vi "test-discretization-14.vi"(8 "error in (no error)":errorcluster) -> (0 "error out":errorcluster, 3 "All Tests Passed":bool)   [LabVIEW 2019]
uses:
  <vilib>/Analysis/Matrix/Datatypes/RealMatrix.ctl
  <vilib>/Analysis/baseanly.llb/Real A x B.vi
  <vilib>/Rock Robotics/WPI/ThirdParty/JAS_Junk/TrajLib/MatBuilder_Create.vi
  <vilib>/Rock Robotics/WPI/ThirdParty/JAS_Junk/TrajLib/MatrixHelper_CoerceSize.vi
  <vilib>/Rock Robotics/WPI/ThirdParty/JAS_Junk/TrajLib/Matrix_Exp.vi
  <vilib>/Rock Robotics/WPI/ThirdParty/JAS_Junk/TrajLib/Matrix_AssignBlock.vi
  <vilib>/Rock Robotics/WPI/ThirdParty/JAS_Junk/TrajLib/Matrix_ExtractFrom.vi
  <vilib>/Analysis/7linalg.llb/Transpose Matrix.vi
  <vilib>/Analysis/7linalg.llb/Real Transpose Matrix.vi
  <vilib>/Rock Robotics/WPI/ThirdParty/JAS_Junk/TrajLib/Matrix_Ident.vi
  <vilib>/Analysis/7linalg.llb/Matrix Exp.vi
  <vilib>/Analysis/7linalg.llb/Real Matrix Exp.vi
  <vilib>/Analysis/Matrix/Numeric/Multiply/Multiply.vi
  <vilib>/Analysis/Matrix/Numeric/Multiply/Multiply - RM,R.vi
  <vilib>/Analysis/7linalg.llb/Create Special Matrix.vi
  <vilib>/Analysis/7linalg.llb/Create Special Real Matrix.vi
  <vilib>/Analysis/Matrix/Numeric/Add/Add - RM,RM.vi
  <vilib>/Analysis/Matrix/Comparison/Equal/Equal - RM,RM.vi
  <vilib>/Rock Robotics/WPI/ThirdParty/JAS_Junk/TrajLib/Trajectory_Library.lvlib
  <vilib>/Analysis/NI_AALBase.lvlib
  <vilib>/Analysis/Matrix/NI_Matrix.lvlib
panel:
  out "X1Discrete 11":T1
  out "DiscB  11":T1
  out "Passed 11":bool
  out "DiscA  11":T1
  out "Passed 10":bool
  out "DiscA  10":T1
  out "Passed 16":bool
  out "DiscR  16":T1
  out "A+B Should be":T1
  out "A + B":T1
  out "Test x passed":bool
  out "Test 3 passed":bool
  out "Test Passed 2":bool
  out "Test Passed 1":bool
  out "Test Passed 0":bool
  out "AQ Passed":bool
  out "AQ - DiscQ":T1
  out "AQ - DiscA":T1
  out "AB-Taylor-Passed":bool
  out "ABTaylor-DiscB":T1
  out "ABTaylor - DiscA":T1
  out "AB-passed":bool
  out "AB-DiscB":T1
  out "AB - DiscA":T1
  out "x1-Disc":T1
  out "DiscA Error":bool
  out "DiscA":T1
  out "Cost Mat":T1
  out "CoVar Mat":T1
  # "1.0,   0.0,    0.0\n\n0.0,     4.0,   0.0, ;\n\n0.0,     0.0,  9.0;"
  # "1.0,      0.0,      0.0, \n\n0.0,   1.0 / 4.0,   0.0, \n\n0.0,       0.0,      1.0 / 9.0,"
  # "VecBuilder.fill(\n          x0.get(0, 0) + 1.0 * x0.get(1, 0), \n          x0.get(1, 0));"
  # "2,\n1"
  # "x0.get(0, 0) + x0.get(1, 0) + 0.5 * u.get(0, 0), \n\nx0.get(0, 0) + u.get(0, 0))"
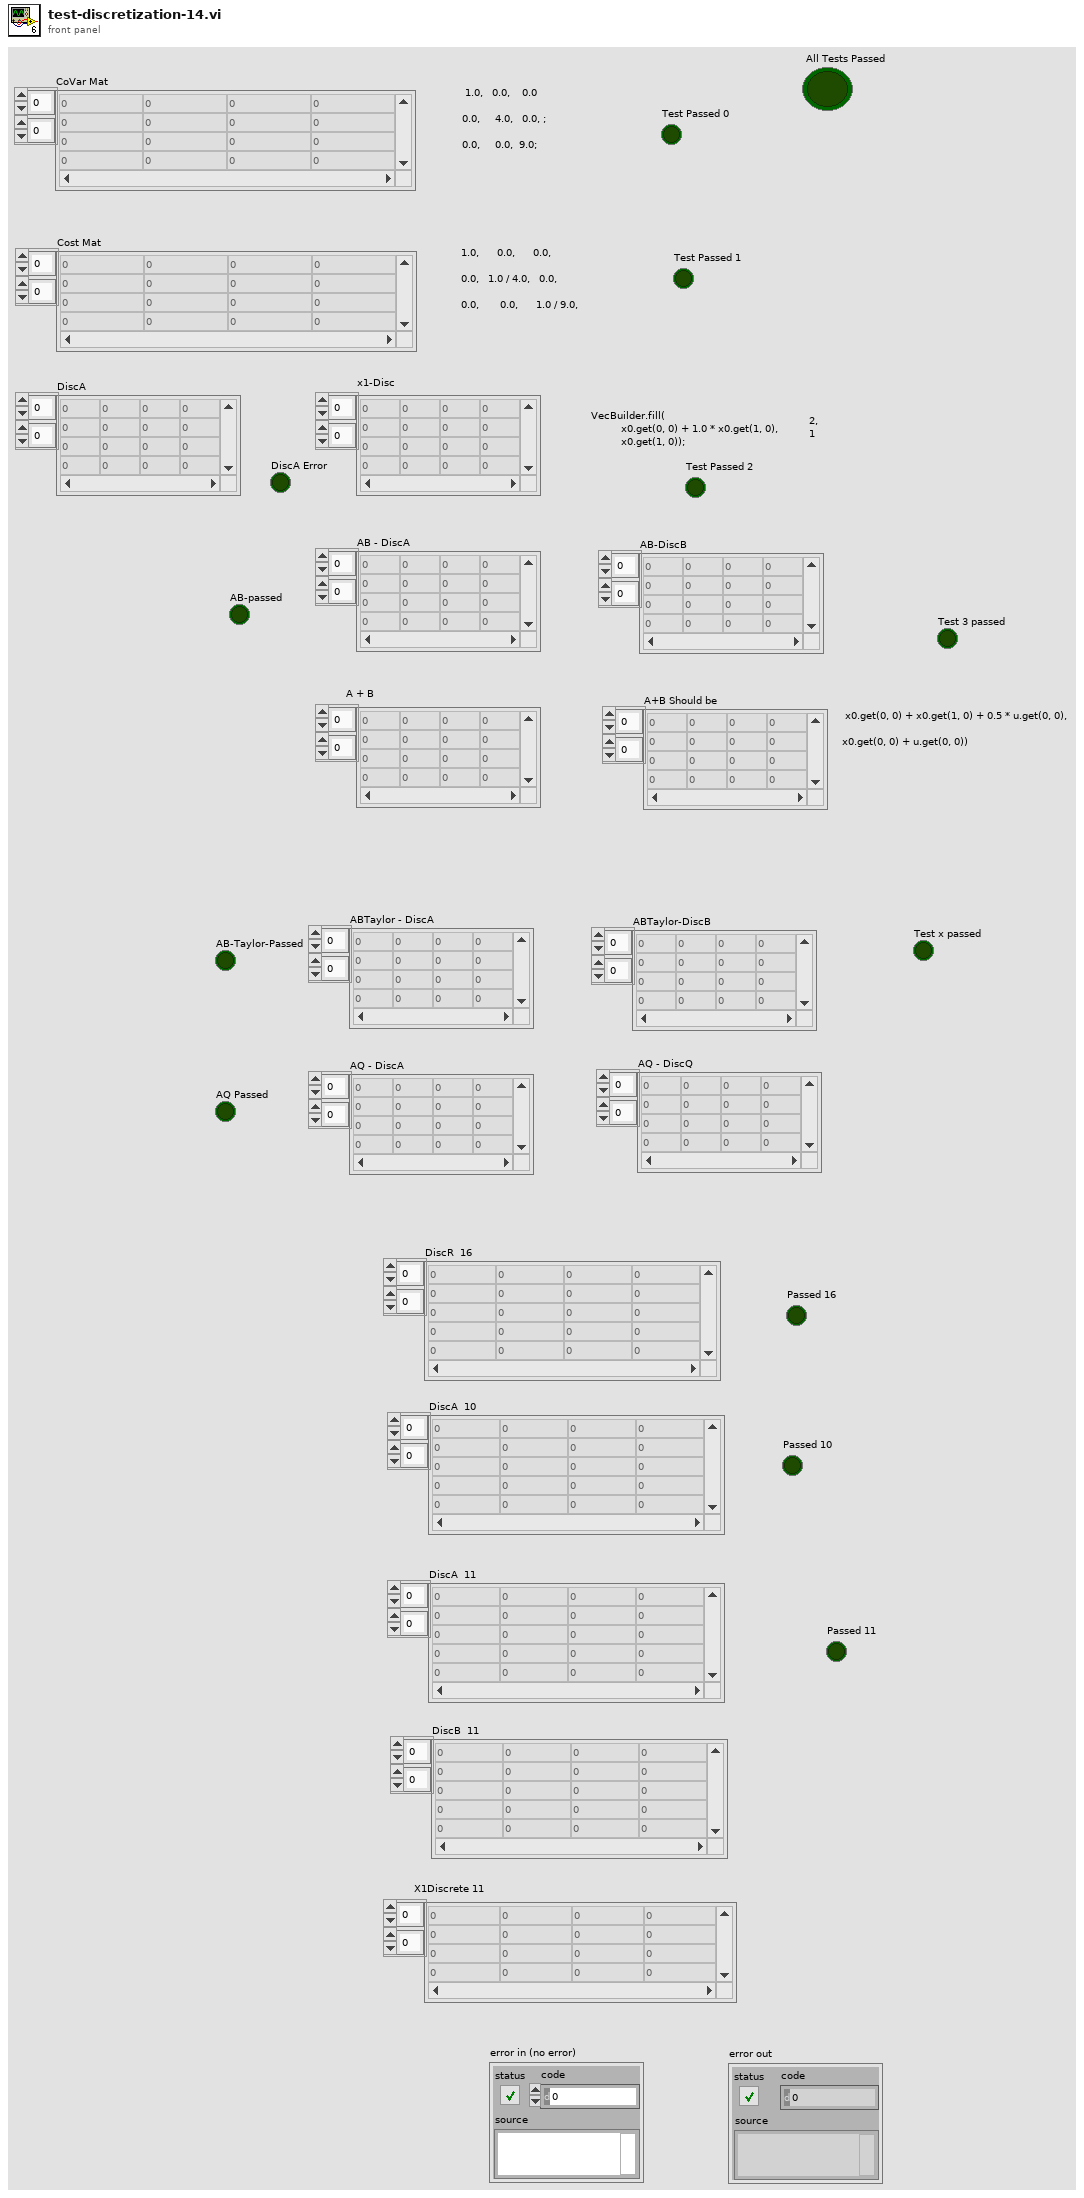
[diagram p1: front panel]
types:
  T1 = typedef "NI_Matrix.lvlib/RealMatrix.ctl" = dbl[][]
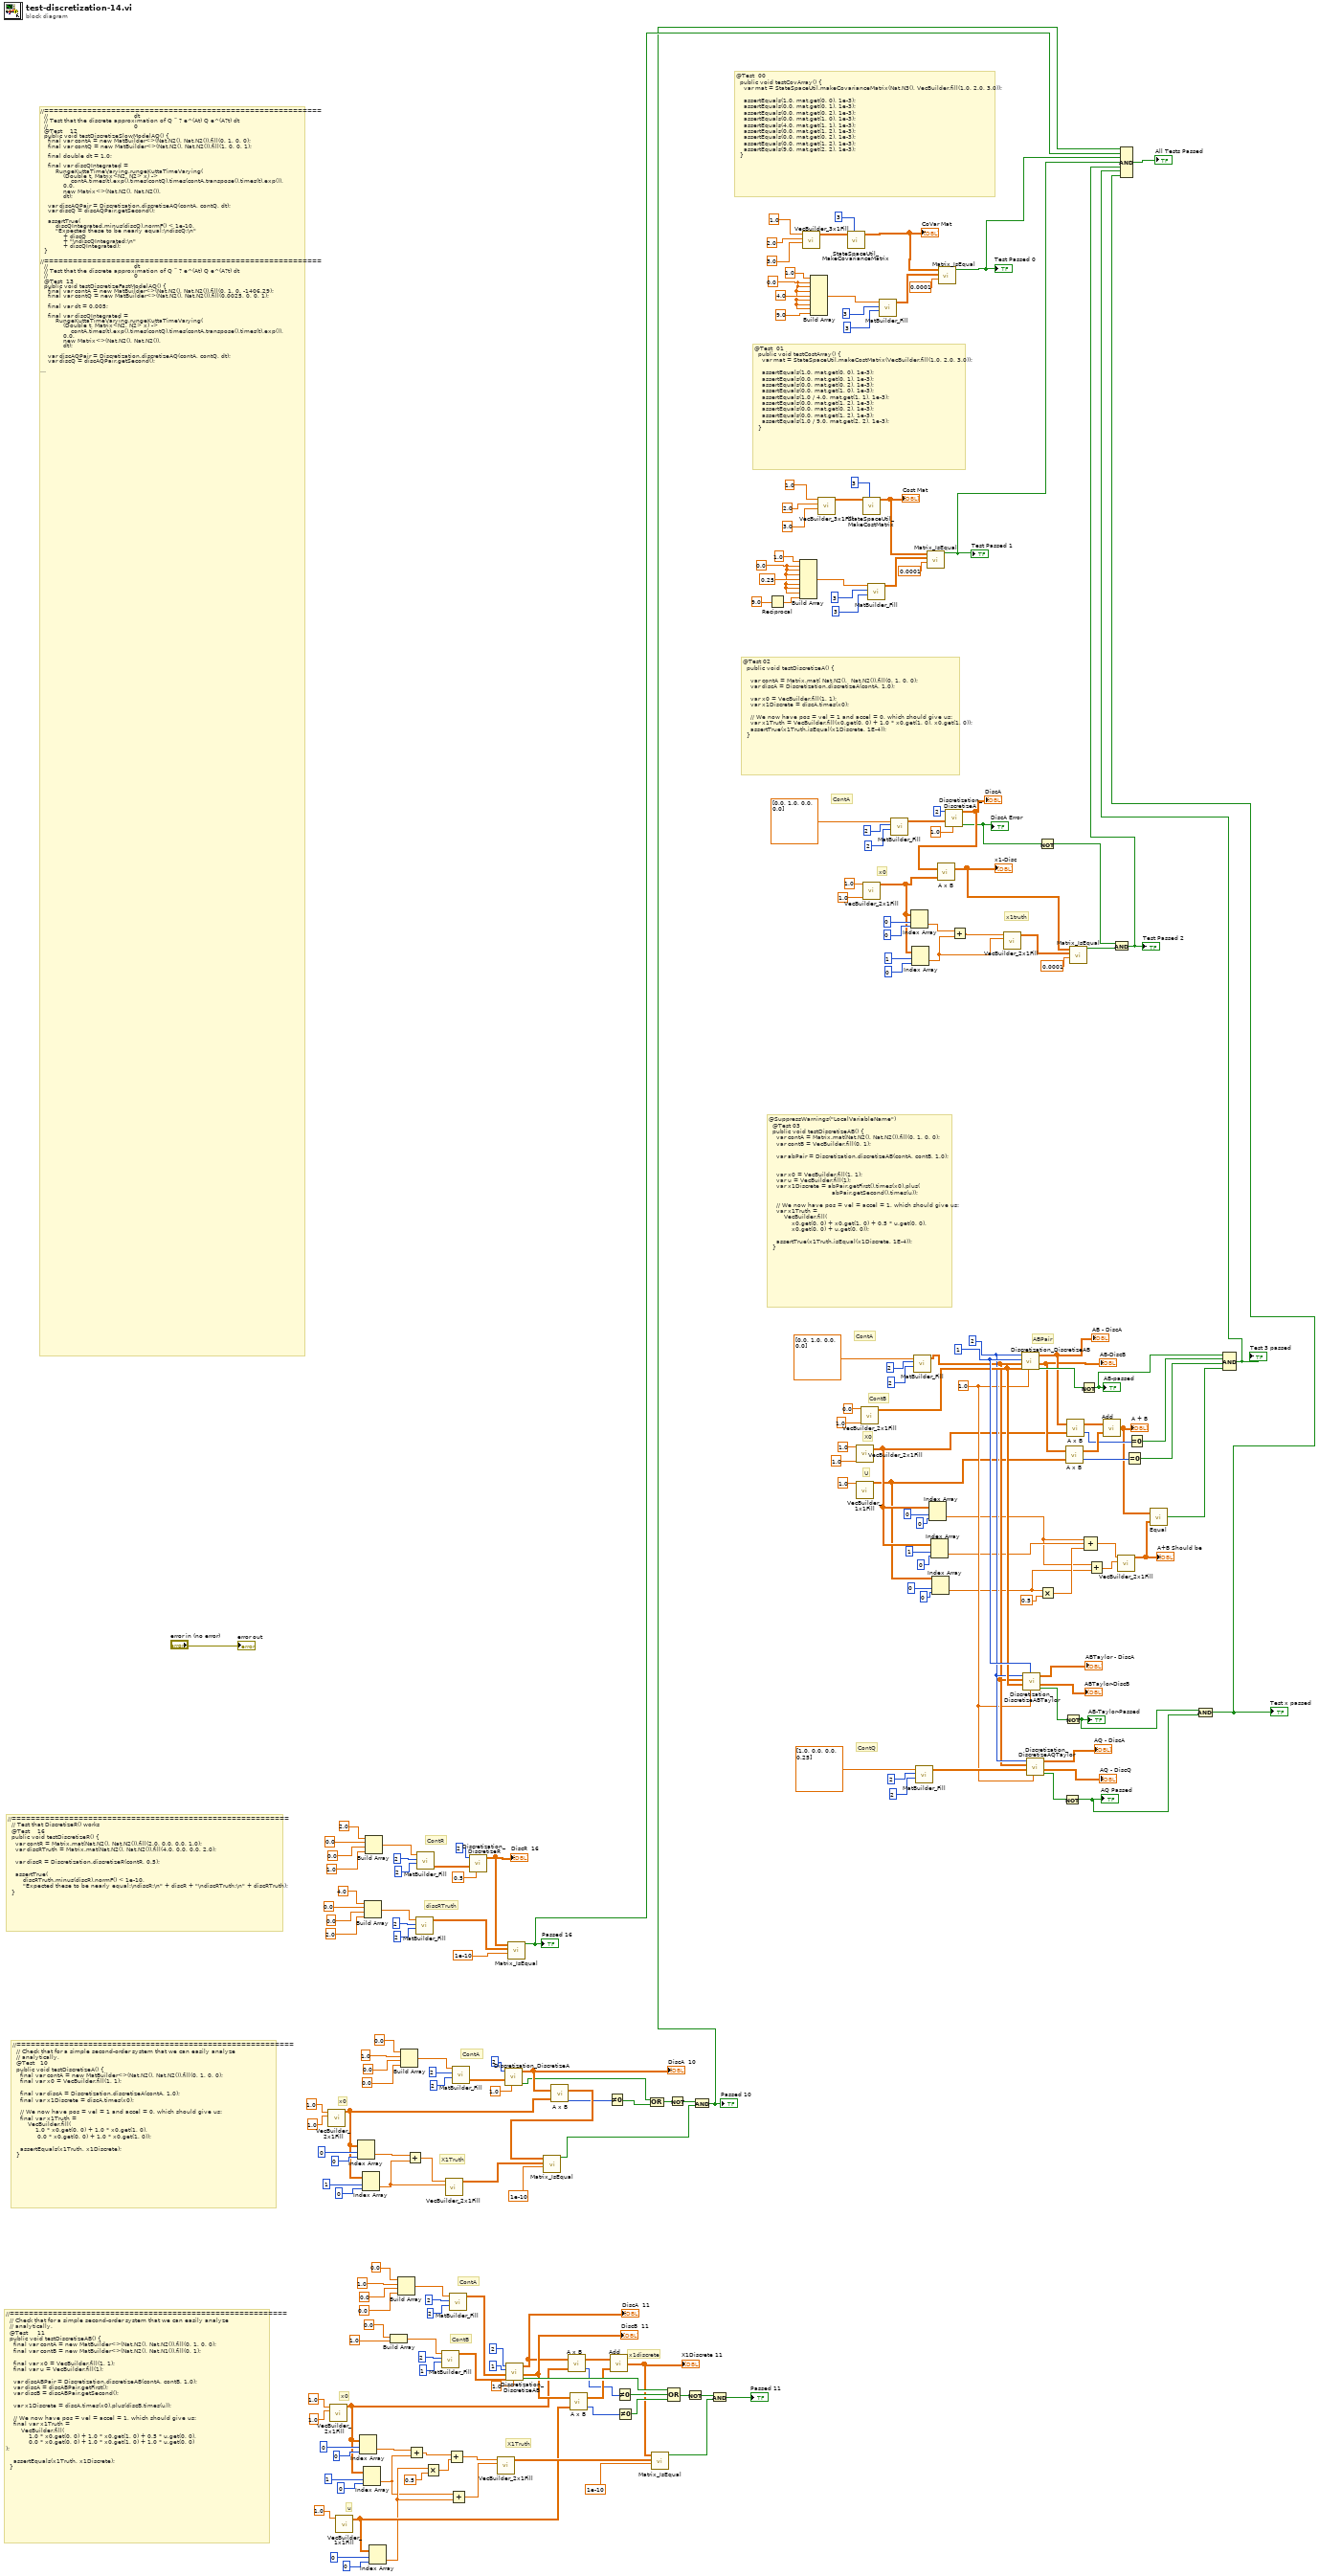
[diagram p0: block diagram]
diagram:
  w166 = 0.0 ("element")
  w176 = 0.0 ("element")
  w184 = 1.0 ("dT_Seconds")
  w194 = 1 ("Inputs")
  w187 = 2 ("States")
  # "x1discrete"
  # "u"
  # "ContB"
  # "X1Truth"
  # "x0"
  # "ContA"
  # "//==========================================================\n  // Check that for a simple second-order system that we can easily analyze\n  // analytically,\n  @Test     11\n  public void testDiscretizeAB() {\n    final var contA = new MatBuilder<>(Nat.N2(), Nat.N2()).fill(0, 1, 0, 0);\n    final var contB = new MatBuilder<>(Nat.N2(), Nat.N1()).fill(0, 1);\n\n    final var x0 = VecBuilder.fill(1, 1);\n    final var u = VecBuilder.fill(1);\n\n    var discABPair = Discretization.discretizeAB(contA, contB, 1.0);\n    var discA = discABPair.getFirst();\n    var discB = discABPair.getSecond();\n\n    var x1Discrete = discA.times(x0).plus(discB.times(u));\n\n    // We now have pos = vel = accel = 1, which should give us:\n    final var x1Truth =\n        VecBuilder.fill(\n            1.0 * x0.get(0, 0) + 1.0 * x0.get(1, 0) + 0.5 * u.get(0, 0),\n            0.0 * x0.get(0, 0) + 1.0 * x0.get(1, 0) + 1.0 * u.get(0, 0)\n);\n\n    assertEquals(x1Truth, x1Discrete);\n  }"
  # "X1Truth"
  # "x0"
  # "ContA"
  # "//==========================================================\n  // Check that for a simple second-order system that we can easily analyze\n  // analytically,\n  @Test   10\n  public void testDiscretizeA() {\n    final var contA = new MatBuilder<>(Nat.N2(), Nat.N2()).fill(0, 1, 0, 0);\n    final var x0 = VecBuilder.fill(1, 1);\n\n    final var discA = Discretization.discretizeA(contA, 1.0);\n    final var x1Discrete = discA.times(x0);\n\n    // We now have pos = vel = 1 and accel = 0, which should give us:\n    final var x1Truth =\n        VecBuilder.fill(\n            1.0 * x0.get(0, 0) + 1.0 * x0.get(1, 0), \n             0.0 * x0.get(0, 0) + 1.0 * x0.get(1, 0));\n\n    assertEquals(x1Truth, x1Discrete);\n  }"
  # "discRTruth"
  # "ContR"
  # "//==========================================================\n  // Test that DiscretizeR() works\n  @Test    16\n  public void testDiscretizeR() {\n    var contR = Matrix.mat(Nat.N2(), Nat.N2()).fill(2.0, 0.0, 0.0, 1.0);\n    var discRTruth = Matrix.mat(Nat.N2(), Nat.N2()).fill(4.0, 0.0, 0.0, 2.0);\n\n    var discR = Discretization.discretizeR(contR, 0.5);\n\n    assertTrue(\n        discRTruth.minus(discR).normF() < 1e-10,\n        \"Expected these to be nearly equal:\\ndiscR:\\n\" + discR + \"\\ndiscRTruth:\\n\" + discRTruth);\n  }"
  # "//==========================================================\n  //                                             dt\n  // Test that the discrete approximation of Q ˜ ? e^(At) Q e^(A?t) dt\n  //                                             0\n  @Test    12\n  public void testDiscretizeSlowModelAQ() {\n    final var contA = new MatBuilder<>(Nat.N2(), Nat.N2()).fill(0, 1, 0, 0);\n    final var contQ = new MatBuilder<>(Nat.N2(), Nat.N2()).fill(1, 0, 0, 1);\n\n    final double dt = 1.0;\n\n    final var discQIntegrated =\n        RungeKuttaTimeVarying.rungeKuttaTimeVarying(\n            (Double t, Matrix<N2, N2> x) ->\n                contA.times(t).exp().times(contQ).times(contA.transpose().times(t).exp()),\n            0.0,\n            new Matrix<>(Nat.N2(), Nat.N2()),\n            dt);\n\n    var discAQPair = Discretization.discretizeAQ(contA, contQ, dt);\n    var discQ = discAQPair.getSecond();\n\n    assertTrue(\n        discQIntegrated.minus(discQ).normF() < 1e-10,\n        \"Expected these to be nearly equal:\\ndiscQ:\\n\"\n            + discQ\n            + \"\\ndiscQIntegrated:\\n\"\n            + discQIntegrated);\n  }\n\n//==========================================================\n  //                                             dt\n  // Test that the discrete approximation of Q ˜ ? e^(At) Q e^(A?t) dt\n  //                                             0\n  @Test  13\n  public void testDiscretizeFastModelAQ() {\n    final var contA = new MatBuilder<>(Nat.N2(), Nat.N2()).fill(0, 1, 0, -1406.29);\n    final var contQ = new MatBuilder<>(Nat.N2(), Nat.N2()).fill(0.0025, 0, 0, 1);\n\n    final var dt = 0.005;\n\n    final var discQIntegrated =\n        RungeKuttaTimeVarying.rungeKuttaTimeVarying(\n            (Double t, Matrix<N2, N2> x) ->\n                contA.times(t).exp().times(contQ).times(contA.transpose().times(t).exp()),\n            0.0,\n            new Matrix<>(Nat.N2(), Nat.N2()),\n            dt);\n\n    var discAQPair = Discretization.discretizeAQ(contA, contQ, dt);\n    var discQ = discAQPair.getSecond();\n\n    assertTrue(\n        discQIntegrated.minus(discQ).normF() < 1e-3,\n        \"Expected these to be nearly equal:\\ndiscQ:\\n\"\n            + discQ\n            + \"\\ndiscQIntegrated:\\n\"\n            + discQIntegrated);\n  }\n\n//==========================================================\n  // Test that the Taylor series discretization produces nearly identical results.\n  @Test  14\n  public void testDiscretizeSlowModelAQTaylor() {\n    final var contA = new MatBuilder<>(Nat.N2(), Nat.N2()).fill(0, 1, 0, 0);\n    final var contQ = new MatBuilder<>(Nat.N2(), Nat.N2()).fill(1, 0, 0, 1);\n\n    final var dt = 1.0;\n\n    // Continuous Q should be positive semidefinite\n    final var esCont = contQ.getStorage().eig();\n    for (int i = 0; i < contQ.getNumRows(); ++i) {\n      assertTrue(esCont.getEigenvalue(i).real >= 0);\n    }\n\n    final var discQIntegrated =\n        RungeKuttaTimeVarying.rungeKuttaTimeVarying(\n            (Double t, Matrix<N2, N2> x) ->\n                contA.times(t).exp().times(contQ).times(contA.transpose().times(t).exp()),\n            0.0,\n            new Matrix<>(Nat.N2(), Nat.N2()),\n            dt);\n\n    var discA = Discretization.discretizeA(contA, dt);\n\n    var discAQPair = Discretization.discretizeAQ(contA, contQ, dt);\n    var discATaylor = discAQPair.getFirst();\n    var discQTaylor = discAQPair.getSecond();\n\n    assertTrue(\n        discQIntegrated.minus(discQTaylor).normF() < 1e-10,\n        \"Expected these to be nearly equal:\\ndiscQTaylor:\\n\"\n            + discQTaylor\n            + \"\\ndiscQIntegrated:\\n\"\n            + discQIntegrated);\n    assertTrue(discA.minus(discATaylor).normF() < 1e-10);\n\n    // Discrete Q should be positive semidefinite\n    final var esDisc = discQTaylor.getStorage().eig();\n    for (int i = 0; i < discQTaylor.getNumRows(); ++i) {\n      assertTrue(esDisc.getEigenvalue(i).real >= 0);\n    }\n  }\n\n//==========================================================\n  // Test that the Taylor series discretization produces nearly identical results.\n  @Test  15\n  public void testDiscretizeFastModelAQTaylor() {\n    final var contA = new MatBuilder<>(Nat.N2(), Nat.N2()).fill(0, 1, 0, -1500);\n    final var contQ = new MatBuilder<>(Nat.N2(), Nat.N2()).fill(0.0025, 0, 0, 1);\n\n    final var dt = 0.005;\n\n    // Continuous Q should be positive semidefinite\n    final var esCont = contQ.getStorage().eig();\n    for (int i = 0; i < contQ.getNumRows(); ++i) {\n      assertTrue(esCont.getEigenvalue(i).real >= 0);\n    }\n\n    final var discQIntegrated =\n        RungeKuttaTimeVarying.rungeKuttaTimeVarying(\n            (Double t, Matrix<N2, N2> x) ->\n                contA.times(t).exp().times(contQ).times(contA.transpose().times(t).exp()),\n            0.0,\n            new Matrix<>(Nat.N2(), Nat.N2()),\n            dt);\n\n    var discA = Discretization.discretizeA(contA, dt);\n\n    var discAQPair = Discretization.discretizeAQ(contA, contQ, dt);\n    var discATaylor = discAQPair.getFirst();\n    var discQTaylor = discAQPair.getSecond();\n\n    assertTrue(\n        discQIntegrated.minus(discQTaylor).normF() < 1e-3,\n        \"Expected these to be nearly equal:\\ndiscQTaylor:\\n\"\n            + discQTaylor\n            + \"\\ndiscQIntegrated:\\n\"\n            + discQIntegrated);\n    assertTrue(discA.minus(discATaylor).normF() < 1e-10);\n\n    // Discrete Q should be positive semidefinite\n    final var esDisc = discQTaylor.getStorage().eig();\n    for (int i = 0; i < discQTaylor.getNumRows(); ++i) {\n      assertTrue(esDisc.getEigenvalue(i).real >= 0);\n    }\n  }\n\n}"
  # "U"
  # "X0"
  # "ContB"
  # "ABPair"
  # "x1truth"
  # "x0"
  # "ContQ"
  # "ContA"
  # "@SuppressWarnings(\"LocalVariableName\")\n  @Test 03\n  public void testDiscretizeAB() {\n    var contA = Matrix.mat(Nat.N2(), Nat.N2()).fill(0, 1, 0, 0);\n    var contB = VecBuilder.fill(0, 1);\n\n    var abPair = Discretization.discretizeAB(contA, contB, 1.0);\n\n\n    var x0 = VecBuilder.fill(1, 1);\n    var u = VecBuilder.fill(1);\n    var x1Discrete = abPair.getFirst().times(x0).plus(\n                                 abPair.getSecond().times(u));\n\n    // We now have pos = vel = accel = 1, which should give us:\n    var x1Truth =\n        VecBuilder.fill(\n            x0.get(0, 0) + x0.get(1, 0) + 0.5 * u.get(0, 0), \n            x0.get(0, 0) + u.get(0, 0));\n\n    assertTrue(x1Truth.isEqual(x1Discrete, 1E-4));\n  }"
  # "ContA"
  # "@Test 02\n  public void testDiscretizeA() {\n\n    var contA = Matrix.mat( Nat.N2(),  Nat.N2()).fill(0, 1, 0, 0);\n    var discA = Discretization.discretizeA(contA, 1.0);\n\n    var x0 = VecBuilder.fill(1, 1);\n    var x1Discrete = discA.times(x0);\n\n    // We now have pos = vel = 1 and accel = 0, which should give us:\n    var x1Truth = VecBuilder.fill(x0.get(0, 0) + 1.0 * x0.get(1, 0), x0.get(1, 0));\n    assertTrue(x1Truth.isEqual(x1Discrete, 1E-4));\n  }"
  # "@Test  01\n  public void testCostArray() {\n    var mat = StateSpaceUtil.makeCostMatrix(VecBuilder.fill(1.0, 2.0, 3.0));\n\n    assertEquals(1.0, mat.get(0, 0), 1e-3);\n    assertEquals(0.0, mat.get(0, 1), 1e-3);\n    assertEquals(0.0, mat.get(0, 2), 1e-3);\n    assertEquals(0.0, mat.get(1, 0), 1e-3);\n    assertEquals(1.0 / 4.0, mat.get(1, 1), 1e-3);\n    assertEquals(0.0, mat.get(1, 2), 1e-3);\n    assertEquals(0.0, mat.get(0, 2), 1e-3);\n    assertEquals(0.0, mat.get(1, 2), 1e-3);\n    assertEquals(1.0 / 9.0, mat.get(2, 2), 1e-3);\n  }"
  # "@Test  00\n  public void testCovArray() {\n    var mat = StateSpaceUtil.makeCovarianceMatrix(Nat.N3(), VecBuilder.fill(1.0, 2.0, 3.0));\n\n    assertEquals(1.0, mat.get(0, 0), 1e-3);\n    assertEquals(0.0, mat.get(0, 1), 1e-3);\n    assertEquals(0.0, mat.get(0, 2), 1e-3);\n    assertEquals(0.0, mat.get(1, 0), 1e-3);\n    assertEquals(4.0, mat.get(1, 1), 1e-3);\n    assertEquals(0.0, mat.get(1, 2), 1e-3);\n    assertEquals(0.0, mat.get(0, 2), 1e-3);\n    assertEquals(0.0, mat.get(1, 2), 1e-3);\n    assertEquals(9.0, mat.get(2, 2), 1e-3);\n  }"
  n1 = call <vilib>:"VecBuilder_2x1Fill.vi"("R1"=1.0, "R0"=1.0) -> ("output matrix"=w66:T1)  [unwired: 9 in]
  n2 = call <vilib>:"VecBuilder_2x1Fill.vi"("R1"=1.0, "R0"=1.0) -> ("output matrix"=w19:T1)  [unwired: 9 in]
  n3 = call <vilib>:"VecBuilder_1x1Fill.vi"("R0_C0"=1.0 ("R0")) -> ("output matrix"=w10:T1)  [unwired: 10 in]
  n4 = Index Array(array=w66, index (row)=0, index (col)=0) -> (element=w63:dbl)
  n5 = Index Array(array=w19, index (row)=0, index (col)=0) -> (element=w37:dbl)
  n6 = Index Array(array=w66, index (row)=1, index (col)=0) -> (element=w62:dbl)
  n7 = Index Array(array=w19, index (row)=1, index (col)=0) -> (element=w4:dbl)
  n8 = Build Array(4.0 ("element"), 0.0 ("element"), 0.0 ("element"), 2.0 ("element")) -> (w98:dbl[])
  n9 = Build Array(2.0 ("element"), 0.0 ("element"), 0.0 ("element"), 1.0 ("element")) -> (w105:dbl[])
  n10 = Index Array(array=w10, index (row)=0, index (col)=0) -> (element=w5:dbl)
  n11 = Build Array(0.0 ("element"), 1.0 ("element")) -> (w30:dbl[])
  n12 = Build Array(0.0 ("element"), 1.0 ("element"), 0.0 ("element"), 0.0 ("element")) -> (w54:dbl[])
  n13 = Build Array(0.0 ("element"), 1.0 ("element"), 0.0 ("element"), 0.0 ("element")) -> (w84:dbl[])
  n14 = Add(x=w63, y=w62) -> (x+y=w64:dbl)
  n15 = Add(x=w37, y=w4) -> (x+y=w7:dbl)
  n16 = call <vilib>:"MatBuilder_Fill.vi"("Columns"=2, "Rows"=2, "Value List"=w98) -> ("output matrix"=w87:T1)  [unwired: 8 in]
  n17 = call <vilib>:"MatBuilder_Fill.vi"("Columns"=2, "Rows"=2, "Value List"=w105) -> ("output matrix"=w90:T1)  [unwired: 8 in]
  n18 = Multiply(x=w5, y=0.5) -> (x*y=w8:dbl)
  n19 = call <vilib>:"MatBuilder_Fill.vi"("Columns"=1, "Rows"=2, "Value List"=w30) -> ("output matrix"=w24:T1)  [unwired: 8 in]
  n20 = call <vilib>:"VecBuilder_2x1Fill.vi"("R1"=w62, "R0"=w64) -> ("output matrix"=w65:T1)  [unwired: 9 in]
  n21 = Add(x=w7, y=w8) -> (x+y=w6:dbl)
  n22 = call <vilib>:"MatBuilder_Fill.vi"("Columns"=2, "Rows"=2, "Value List"=w54) -> ("output matrix"=w25:T1)  [unwired: 8 in]
  n23 = Add(x=w4, y=w5) -> (x+y=w3:dbl)
  n24 = call <vilib>:"MatBuilder_Fill.vi"("Columns"=2, "Rows"=2, "Value List"=w84) -> ("output matrix"=w76:T1)  [unwired: 8 in]
  n25 = call <vilib>:"Discretization_DiscretizeR.vi"("dT_Seconds"=0.5, "ContR"=w90, "Outputs"=2) -> ("DiscR"=w89:T1)  [unwired: 7 in, 1 out]
  "DiscR  16" <- w89
  n26 = call <vilib>:"VecBuilder_2x1Fill.vi"("R1"=w3, "R0"=w6) -> ("output matrix"=w38:T1)  [unwired: 9 in]
  n27 = call <vilib>:"Discretization_DiscretizeA.vi"("dT_Seconds"=1.0, "ContA"=w76, "States"=2 ("Outputs")) -> ("Error"=w59:bool, "DiscA"=w71:T1)  [unwired: 7 in]
  "DiscA  10" <- w71
  n28 = call <vilib>:"Discretization_DiscretizeAB.vi"("dT_Seconds"=1.0, "ContB"=w24, "ContA"=w25, "Inputs"=1, "States"=2 ("Outputs")) -> ("Error"=w36:bool, "DiscB"=w21:T1, "DiscA"=w20:T1)  [unwired: 4 in]
  "DiscA  11" <- w20
  "DiscB  11" <- w21
  n29 = call <vilib>:"Matrix_IsEqual.vi"("Tolerance"=1e-10, "other"=w87, "input matrix"=w89) -> ("Equal"=w85:bool)  [unwired: 8 in]
  "Passed 16" <- w85
  n30 = call-poly <vilib>:"A x B.vi"("B"=w66, "A"=w71) -> ("error"=w60:i32, "A x B"=w61:T1)
  n31 = call <vilib>:"Matrix_IsEqual.vi"("Tolerance"=1e-10, "other"=w65, "input matrix"=w61) -> ("Equal"=w55:bool)  [unwired: 8 in]
  n32 = call-poly <vilib>:"A x B.vi"("B"=w19, "A"=w20) -> ("error"=w15:i32, "A x B"=w18:T1)
  n33 = call-poly <vilib>:"A x B.vi"("B"=w10, "A"=w21) -> ("error"=w14:i32, "A x B"=w17:T1)
  n34 = Not Equal To 0?(x=w60) -> (x != 0?=w58:bool)
  n35 = call-poly <vilib>:"Add.vi"("Real Matrix B"=w17, "Real Matrix A"=w18) -> ("A + B"=w13:T1)
  "X1Discrete 11" <- w13
  n36 = Not Equal To 0?(x=w15) -> (x != 0?=w35:bool)
  n37 = Not Equal To 0?(x=w14) -> (x != 0?=w16:bool)
  n38 = Compound Arithmetic op=OR(w59, w58) -> (w57:bool)
  n39 = call <vilib>:"Matrix_IsEqual.vi"("Tolerance"=1e-10, "other"=w38, "input matrix"=w13) -> ("Equal"=w32:bool)  [unwired: 8 in]
  n40 = Compound Arithmetic op=OR(w36, w35, w16) -> (w34:bool)
  n41 = Not(x=w57) -> (.not. x?=w56:bool)
  n42 = Not(x=w34) -> (.not. x?=w33:bool)
  n43 = And(x=w56, y=w55) -> (x .and. y?=w2:bool)
  "Passed 10" <- w2
  n44 = And(x=w33, y=w32) -> (x .and. y?=→"Passed 11":bool)
  n45 = Reciprocal(x=9.0 ("element")) -> (1/x=w162:dbl)
  n46 = Build Array(1.0 ("element"), w166, w166, w166, 0.25 ("element"), w166, w166, w166, w162) -> (w169:dbl[])
  n47 = call <vilib>:"VecBuilder_3x1Fill.vi"("R2"=3.0, "R1"=2.0, "R0"=1.0) -> ("output matrix"=w215:T1)  [unwired: 8 in]
  n48 = Build Array(1.0 ("element"), w176, w176, w176, 4.0 ("element"), w176, w176, w176, 9.0 ("element")) -> (w179:dbl[])
  n49 = call <vilib>:"VecBuilder_3x1Fill.vi"("R2"=3.0, "R1"=2.0, "R0"=1.0) -> ("output matrix"=w210:T1)  [unwired: 8 in]
  n50 = call <vilib>:"StateSpaceUtil_MakeCovarianceMatrix.vi"("States"=3, "StdDevs"=w215) -> ("Covariance Matrix"=w174:T1)  [unwired: 8 in, 1 out]
  "CoVar Mat" <- w174
  n51 = call <vilib>:"VecBuilder_2x1Fill.vi"("R1"=1.0, "R0"=1.0 ("R0_C0")) -> ("output matrix"=w117:T1)  [unwired: 9 in]
  n52 = call <vilib>:"VecBuilder_1x1Fill.vi"("R0_C0"=1.0) -> ("output matrix"=w116:T1)  [unwired: 10 in]
  n53 = call <vilib>:"VecBuilder_2x1Fill.vi"("R1"=1.0, "R0"=0.0 ("R0_C0")) -> ("output matrix"=w193:T1)  [unwired: 9 in]
  n54 = call <vilib>:"StateSpaceUtil_MakeCostMatrix.vi"("States"=3, "Costs"=w210) -> ("Costs Matrix"=w161:T1)  [unwired: 8 in, 1 out]
  "Cost Mat" <- w161
  n55 = call <vilib>:"VecBuilder_2x1Fill.vi"("R1"=1.0, "R0"=1.0 ("R0_C0")) -> ("output matrix"=w155:T1)  [unwired: 9 in]
  n56 = call <vilib>:"MatBuilder_Fill.vi"("Columns"=3, "Rows"=3, "Value List"=w169) -> ("output matrix"=w165:T1)  [unwired: 8 in]
  n57 = call <vilib>:"MatBuilder_Fill.vi"("Columns"=3, "Rows"=3, "Value List"=w179) -> ("output matrix"=w173:T1)  [unwired: 8 in]
  n58 = call <vilib>:"MatBuilder_Fill.vi"("Columns"=2, "Rows"=2, "Value List"=dbl[] [0.0, 1.0, 0.0, 0.0]) -> ("output matrix"=w203:T1)  [unwired: 8 in]
  n59 = Index Array(array=w155, index (row)=0, index (col)=0) -> (element=w154:dbl)
  n60 = Index Array(array=w155, index (row)=1, index (col)=0) -> (element=w152:dbl)
  n61 = call <vilib>:"MatBuilder_Fill.vi"("Columns"=2, "Rows"=2, "Value List"=dbl[] [0.0, 1.0, 0.0, 0.0]) -> ("output matrix"=w186:T1)  [unwired: 8 in]
  n62 = call <vilib>:"MatBuilder_Fill.vi"("Columns"=2, "Rows"=2, "Value List"=dbl[] [1.0, 0.0, 0.0, 0.25]) -> ("output matrix"=w185:T1)  [unwired: 8 in]
  n63 = call <vilib>:"Matrix_IsEqual.vi"("Tolerance"=0.0001, "other"=w165, "input matrix"=w161) -> ("Equal"=w145:bool)  [unwired: 8 in]
  "Test Passed 1" <- w145
  n64 = Index Array(array=w117, index (row)=0, index (col)=0) -> (element=w110:dbl)
  n65 = Index Array(array=w117, index (row)=1, index (col)=0) -> (element=w114:dbl)
  n66 = Index Array(array=w116, index (row)=0, index (col)=0) -> (element=w109:dbl)
  n67 = call <vilib>:"Matrix_IsEqual.vi"("Tolerance"=0.0001, "other"=w173, "input matrix"=w174) -> ("Equal"=w146:bool)  [unwired: 8 in]
  "Test Passed 0" <- w146
  n68 = call <vilib>:"Discretization_DiscretizeA.vi"("dT_Seconds"=1.0, "ContA"=w203, "States"=2) -> ("Error"=w148:bool, "DiscA"=w200:T1)  [unwired: 7 in]
  "DiscA" <- w200
  "DiscA Error" <- w148
  n69 = call-poly <vilib>:"A x B.vi"("B"=w155, "A"=w200) -> ("A x B"=w151:T1)  [unwired: 1 out]
  "x1-Disc" <- w151
  n70 = Add(x=w154, y=w152) -> (x+y=w153:dbl)
  n71 = call <vilib>:"VecBuilder_2x1Fill.vi"("R1"=w152, "R0"=w153) -> ("output matrix"=w150:T1)  [unwired: 9 in]
  n72 = call <vilib>:"Discretization_DiscretizeAB.vi"("dT_Seconds"=w184, "ContB"=w193, "ContA"=w186, "Inputs"=w194, "States"=w187) -> ("Error"=w142:bool, "DiscB"=w132:T1, "DiscA"=w136:T1)  [unwired: 4 in]
  "AB - DiscA" <- w136
  "AB-DiscB" <- w132
  n73 = call <vilib>:"Discretization_DiscretizeABTaylor.vi"("dT_Seconds"=w184, "Inputs"=w194, "ContB"=w193, "ContA"=w186, "States"=w187) -> ("Error"=w141:bool, "DiscB"=→"ABTaylor-DiscB":T1, "DiscA"=→"ABTaylor - DiscA":T1)  [unwired: 4 in]
  n74 = call <vilib>:"Discretization_DiscretizeAQTaylor.vi"("dT_Seconds"=w184, "ContQ"=w185, "ContA"=w186, "States"=w187) -> ("Error"=w139:bool, "DiscQ"=→"AQ - DiscQ":T1, "DiscA"=→"AQ - DiscA":T1)  [unwired: 5 in]
  n75 = Not(x=w148) -> (.not. x?=w147:bool)
  n76 = Multiply(x=w109, y=0.5) -> (x*y=w113:dbl)
  n77 = Not(x=w139) -> (.not. x?=w137:bool)
  "AQ Passed" <- w137
  n78 = Not(x=w141) -> (.not. x?=w138:bool)
  "AB-Taylor-Passed" <- w138
  n79 = call-poly <vilib>:"A x B.vi"("B"=w116, "A"=w132) -> ("error"=w128:i32, "A x B"=w130:T1)
  n80 = call-poly <vilib>:"A x B.vi"("B"=w117, "A"=w136) -> ("error"=w129:i32, "A x B"=w131:T1)
  n81 = call <vilib>:"Matrix_IsEqual.vi"("Tolerance"=0.0001, "other"=w150, "input matrix"=w151) -> ("Equal"=w149:bool)  [unwired: 8 in]
  n82 = Not(x=w142) -> (.not. x?=w140:bool)
  "AB-passed" <- w140
  n83 = Compound Arithmetic op=ADD(w110, w114, w113) -> (w112:dbl)
  n84 = Add(x=w110, y=w109) -> (x+y=w111:dbl)
  n85 = call-poly <vilib>:"Add.vi"("Real Matrix B"=w130, "Real Matrix A"=w131) -> ("A + B"=w107:T1)
  "A + B" <- w107
  n86 = Compound Arithmetic op=AND(w147, w149) -> (w144:bool)
  "Test Passed 2" <- w144
  n87 = call <vilib>:"VecBuilder_2x1Fill.vi"("R1"=w111, "R0"=w112) -> ("output matrix"=w108:T1)  [unwired: 9 in]
  "A+B Should be" <- w108
  n88 = Equal To 0?(x=w128) -> (x = 0?=w126:bool)
  n89 = Equal To 0?(x=w129) -> (x = 0?=w127:bool)
  n90 = call-poly <vilib>:"Equal.vi"("Real Matrix B"=w108, "Real Matrix A"=w107) -> ("A = B?"=w106:bool)
  n91 = Compound Arithmetic op=AND(w138, w137) -> (w124:bool)
  "Test x passed" <- w124
  n92 = Compound Arithmetic op=AND(w140, w127, w126, w106) -> (w125:bool)
  "Test 3 passed" <- w125
  n93 = Compound Arithmetic op=AND(w2, w85, w146, w145, w144, w125, w124) -> (→"All Tests Passed":bool)
  "error out" <- "error in (no error)"
